vi "ResMgr-Request lvlibp Minimum Version.vi"(6 "Timeout In ms (5000 ms)":i32=5000, 8 "Error In":errorcluster caption="error in (no error)") -> (0 "error out":errorcluster, 3 "CSM Version":T1)   [LabVIEW 2017, in "Communicable State Machine.lvlib"]
uses:
  Communicable State Machine.lvlib
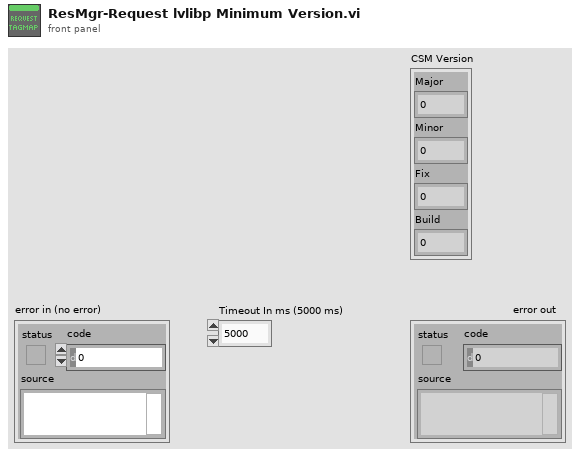
[diagram p1: front panel]
types:
  T1 = cluster{"Major":u16, "Minor":u16, "Fix":u16, "Build":u16}
  T2 = cluster{"ResType":string, "RespQ":refnum<queue>, "Parameter":string, "WatchDogQ":refnum<queue>}
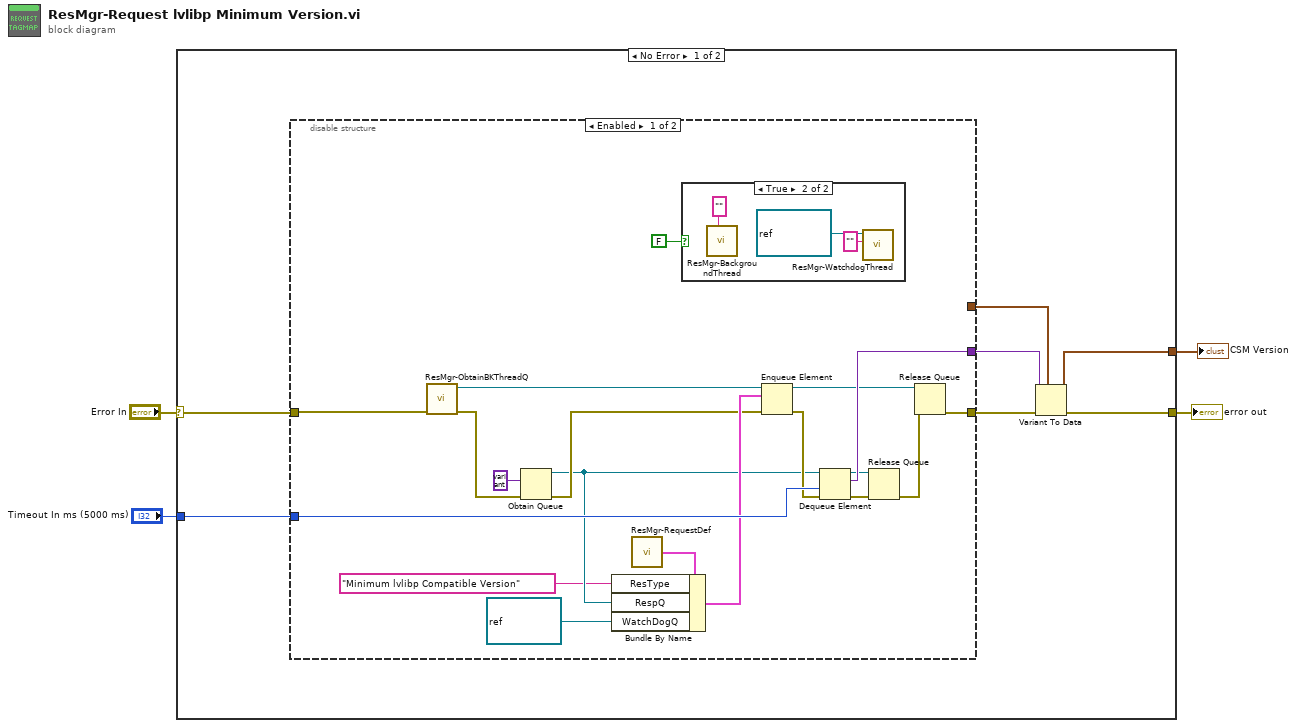
[diagram p0: block diagram]
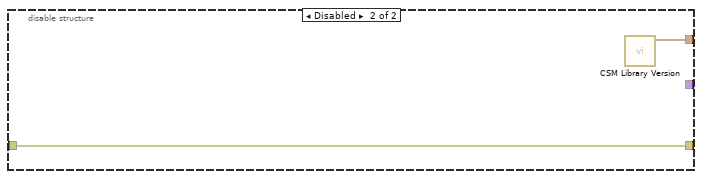
[diagram p3: hidden frame]
diagram:
  n1 = case shown="No Error" "Error In" {
    selector: "Error In" -> [w10 w36]
    tunnel: [w9 w36] -> w4
    tunnel: [w8 _] -> w1
    tunnel: "Timeout In ms (5000 ms)" -> [w11 _]
    frame No Error {
      n2 = disable-structure shown="Enabled" {
        disable-tunnel: [w30 w35] -> w7
        disable-tunnel: w11 -> [w29 _]
        disable-tunnel: [w28 _] -> w6
        disable-tunnel: w10 -> [w14 w35]
        disable-tunnel: [_ w34] -> w5
        frame Enabled {
          n3 = call "ResMgr-ObtainBKThreadQ.vi"("error in (no error)"=w14) -> ("error out"=w15:errorcluster, "ObtainBKThreadQ"=w16:refnum<queue>)  [unwired: 9 in]
          n4 = Obtain Queue(element data type=variant, error in (no error)=w15) -> (queue out=w18:refnum<queue>, error out=w26:errorcluster)  [unwired: 3 in, 1 out]
          n5 = call "ResMgr-RequestDef.vi"() -> ("ResMgr-RequestDef.ctl"=w13:T2)  [unwired: 2 in]
          n6 = Bundle By Name(cluster=w13, "ResType"="Minimum lvlibp Compatible Version", "RespQ"=w18, "WatchDogQ"=refnum<queue> refnum) -> (w27:T2)
          n7 = case shown="True" FALSE {
            frame False {
            }
            frame True {
              n8 = call "ResMgr-BackgroundThread.vi"("Name (Unnamed)"="" ("name (unnamed)")) -> ()  [unwired: 11 in]
              n9 = call "ResMgr-WatchdogThread.vi"("From Who"="", "WatchDogQ"=refnum<queue> refnum) -> ()  [unwired: 10 in]
            }
          }
          n10 = Enqueue Element(queue=w16, element=w27, error in (no error)=w26) -> (queue out=w22:refnum<queue>, error out=w25:errorcluster)  [unwired: 1 in, 1 out]
          n11 = Dequeue Element(queue=w18, timeout in ms (-1)=w29, error in (no error)=w25) -> (queue out=w23:refnum<queue>, element=w28:variant, error out=w24:errorcluster)  [unwired: 1 out]
          n12 = Release Queue(queue=w23, error in (no error)=w24) -> (error out=w21:errorcluster)  [unwired: 1 in, 2 out]
          n13 = Release Queue(queue=w22, error in (no error)=w21) -> (error out=w30:errorcluster)  [unwired: 1 in, 2 out]
        }
        frame Disabled {
          n14 = call "CSM Library Version.vi"() -> ("Min-Compatible Version"=w34:T1)  [unwired: 10 in, 1 out]
        }
      }
      n15 = Variant To Data(error in=w7, type=w5, Variant=w6) -> (data=w8:T1, error out=w9:errorcluster)
    }
    frame Error {
    }
  }
  "error out" <- w4
  "CSM Version" <- w1
